vi "RSZVB Set Pulse Generator Single Period.vi"(8 "error in (no error)":errorcluster {"code" format="%.0x"}, 9 "Single Pulse Period (100.0e-6 s)":dbl=0.0001 format="%^.3e", 10 "Channel (1)":i32=1, 11 "VISA session":refnum<visa-resource-name>) -> (0 "error out":errorcluster {"code" format="%.0x"}, 3 "dup VISA session":refnum<visa-resource-name>)   [LabVIEW 2011]
doc: "This VI defines the pulse period of the single pulse generator signal. \n\nNote(s):\n\n(1) This VI is available only with option R&S ZVA-K27.\n\nRemote-control command(s):\n[SENSe<Ch>:]PULSe:GENerator<gen_no>:PERiod"
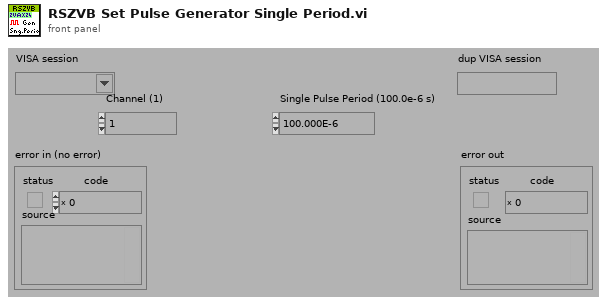
[diagram p1: front panel]
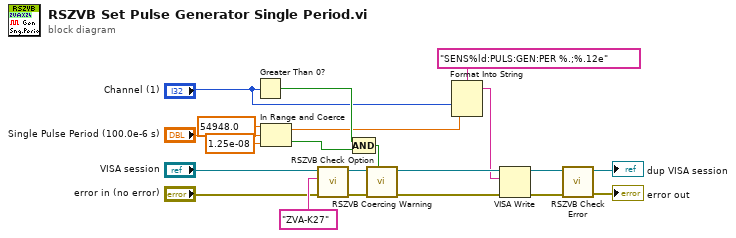
[diagram p0: block diagram]
diagram:
  n1 = Greater Than 0?(x="Channel (1)") -> (x > 0?=w8:bool)
  n2 = In Range and Coerce(upper limit=54948.0, x="Single Pulse Period (100.0e-6 s)", lower limit=1.25e-08) -> (coerced(x)=w3:dbl, In Range?=w9:bool)
  n3 = call "RSZVB Check Option.vi"("error in (no error)"="error in (no error)", "Options"="ZVA-K27", "VISA session"="VISA session") -> ("error out"=w15:errorcluster, "dup VISA session"=w14:refnum<visa-resource-name>)  [unwired: 7 in]
  n4 = Compound Arithmetic op=AND(w8, w9) -> (w11:bool)
  n5 = call "RSZVB Coercing Warning.vi"("In Range?"=w11, "error in (no error)"=w15, "VISA session"=w14) -> ("error out"=w20:errorcluster, "dup VISA session"=w21:refnum<visa-resource-name>)  [unwired: 7 in]
  n6 = Format Into String(format string="SENS%ld:PULS:GEN:PER %.;%.12e", "Channel (1)", w3) -> (resulting string=w17:string)  [unwired: 2 in, 1 out]
  n7 = VISA Write(VISA resource name=w21, write buffer=w17, error in (no error)=w20) -> (VISA resource name out=w18:refnum<visa-resource-name>, error out=w19:errorcluster)  [unwired: 1 out]
  n8 = call "RSZVB Check Error.vi"("error in (no error)"=w19, "VISA session"=w18) -> ("error out"=→"error out":errorcluster, "dup VISA session"=→"dup VISA session":refnum<visa-resource-name>)  [unwired: 8 in]
